vi "Teleop.vi"(10 "Match Info":T1={"Autonomous Elapsed Seconds"=0.0, "TeleOp Elapsed Seconds"=0.0, "Disabled Elapsed Seconds"=0.0, "Visited Autonomous"=FALSE, "Visited TeleOp"=FALSE, "Visited Disabled"=FALSE, "Autonomous Settings"={"Autonomous Style"=enum."Independent", "VI Refnum"=refnum}}, 11 "Call Context":T2) -> ()   [LabVIEW 2020]
doc: "This VI is called for each TeleOp packet received from the DS where the robot is not disabled. It is often used to read from the joysticks and update I/O or to update setpoints for timed control loops. It should complete and return within 20 milliseconds or it may miss DS packets."
uses:
  <vilib>/Rock Robotics/WPI/DriverStation/WPI_DriverStationDerivedRobotMode.ctl
  <vilib>/Rock Robotics/WPI/DriverStation/WPI_DriverStationMatch Info.ctl
  <vilib>/Rock Robotics/WPI/Joystick/XBox Axes Indexer.ctl
  <vilib>/Rock Robotics/WPI/ThirdParty/Phoenix-LabVIEW/Motor Controller/Controls/CTRE_Phoenix_MotorControl_ControlMode.ctl
  <vilib>/Rock Robotics/WPI/Utilities/WPI_GetSetVariantRefNum.vi
  <vilib>/Rock Robotics/Network Tables/NT Write Boolean Array.vi
  <vilib>/Rock Robotics/Network Tables/NT Write Numeric Array.vi
  <vilib>/Rock Robotics/Network Tables/NT Read Boolean.vi
  <vilib>/Rock Robotics/Network Tables/NT Read Number.vi
  <vilib>/Rock Robotics/WPI/ThirdParty/Phoenix-LabVIEW/Motor Controller/Get/CTRE_Phoenix_MotorController_GetSelectedSensorData.vi
panel:
  out "Voltage":dbl
  out "Sample Slider 0":dbl(slide) scale=0.0..5.0
  out "Sample Boolean 1":bool
  out "Sample Boolean 0":bool
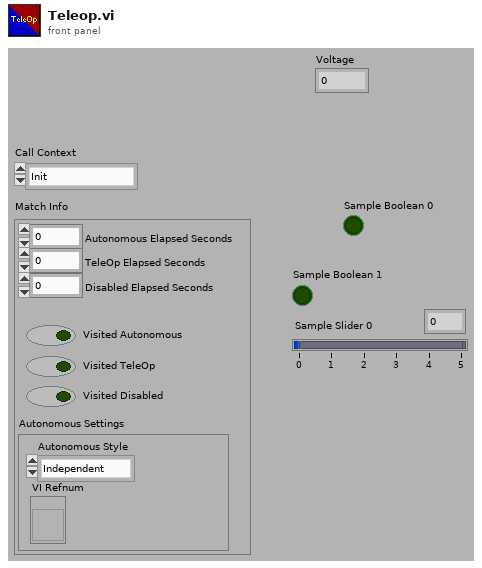
[diagram p1: front panel]
types:
  T1 = typedef "WPI_DriverStationMatch Info.ctl" = cluster{"Autonomous Elapsed Seconds":dbl, "TeleOp Elapsed Seconds":dbl, "Disabled Elapsed Seconds":dbl, "Visited Autonomous":bool, "Visited TeleOp":bool, "Visited Disabled":bool, "Autonomous Settings":cluster{"Autonomous Style":enum16{"Iterative", "Independent"}, "VI Refnum":refnum<vi>}}
  T2 = typedef "WPI_DriverStationDerivedRobotMode.ctl" = enum16{"Init", "Execute", "Stop"}
  T3 = typedef "CTRE_Phoenix_MotorControl_ControlMode.ctl" = u16
  T4 = typedef "XBox Axes Indexer.ctl" = enum16{"Left X", "Left Y", "Left Trigger", "Right Trigger", "Right X", "Right Y"}
  T5 = typedef "WPI_AnalogChannelDevRef.ctl" = cluster{"DevStatus":errorcluster, "Analog Channel":T6}
  T6 = typedef "FPGA_AIChannel.ctl" = enum8{"AI 0", "AI 1", "AI 2", "AI 3", "AI MXP 0", "AI MXP 1", "AI MXP 2", "AI MXP 3", "Invalid"}
  T7 = typedef "WPI_RobotDriveDevRef.ctl" = cluster{"DevStatus":errorcluster, "Motors[]":T8[], "Square Inputs":bool, "Max Output":dbl}
  T8 = typedef "WPI_MotorControlDeviceRef.ctl" = cluster{"DeviceStatus":errorcluster, "Type":T9, "PWM":cluster{"PWM Channel":T10, "DeadBand":T11}, "CAN":cluster{"Device Number":u8, "SetOutput VI Ref":variant, "GetOutput VI Ref":variant, "Enable VI Ref":variant, "Disable VI Ref":variant, "Data":variant}, "Invert":bool, "DIO PWM":cluster{"PWM \"Enable\" Channel":T10, "DIOChannel":T12, "PWM Rate":dbl}}
  T9 = typedef "WPI_MotorControlType.ctl" = enum16{"PWM", "CAN", "DIO PWM"}
  T10 = typedef "FPGA_DIOPWMChannel.ctl" = enum8{"PWM 0", "PWM 1", "PWM 2", "PWM 3", "PWM 4", "PWM 5", "PWM 6", "PWM 7", "PWM 8", "PWM 9", "PWM MXP 0", "PWM MXP 1", "PWM MXP 2", "PWM MXP 3", "PWM MXP 4", "PWM MXP 5", "PWM MXP 6", "PWM MXP 7", "PWM MXP 8", "PWM MXP 9", "Invalid"}
  T11 = typedef "WPI_PWMDeadband.ctl" = cluster{"Name":string, "maxPositivePwm":i32, "minPositivePwm":i32, "centerPwm":i32, "maxNegativePwm":i32, "minNegativePwm":i32, "angularRange":u16}
  T12 = typedef "FPGA_DIOChannel.ctl" = enum8{"DIO 0", "DIO 1", "DIO 2", "DIO 3", "DIO 4", "DIO 5", "DIO 6", "DIO 7", "DIO 8", "DIO 9", "DIO MXP 0", "DIO MXP 1", "DIO MXP 2", "DIO MXP 3", "DIO MXP 4", "DIO MXP 5", "DIO MXP 6", "DIO MXP 7", "DIO MXP 8", "DIO MXP 9", "DIO MXP 10", "DIO MXP 11", "DIO MXP 12", "DIO MXP 13", "DIO MXP 14", "DIO MXP 15", "SPI Port CS1", "SPI Port CS2", "SPI Port CS3", "SPI Port MISO", "SPI Port MOSI", "Invalid"}
  T13 = typedef "WPI_JoystickDevRef.ctl" = cluster{"Device":T14}
  T14 = typedef "WPI_JoystickDeviceEnum.ctl" = enum16{"USB 0", "USB 1", "USB 2", "USB 3", "USB 4", "USB 5"}
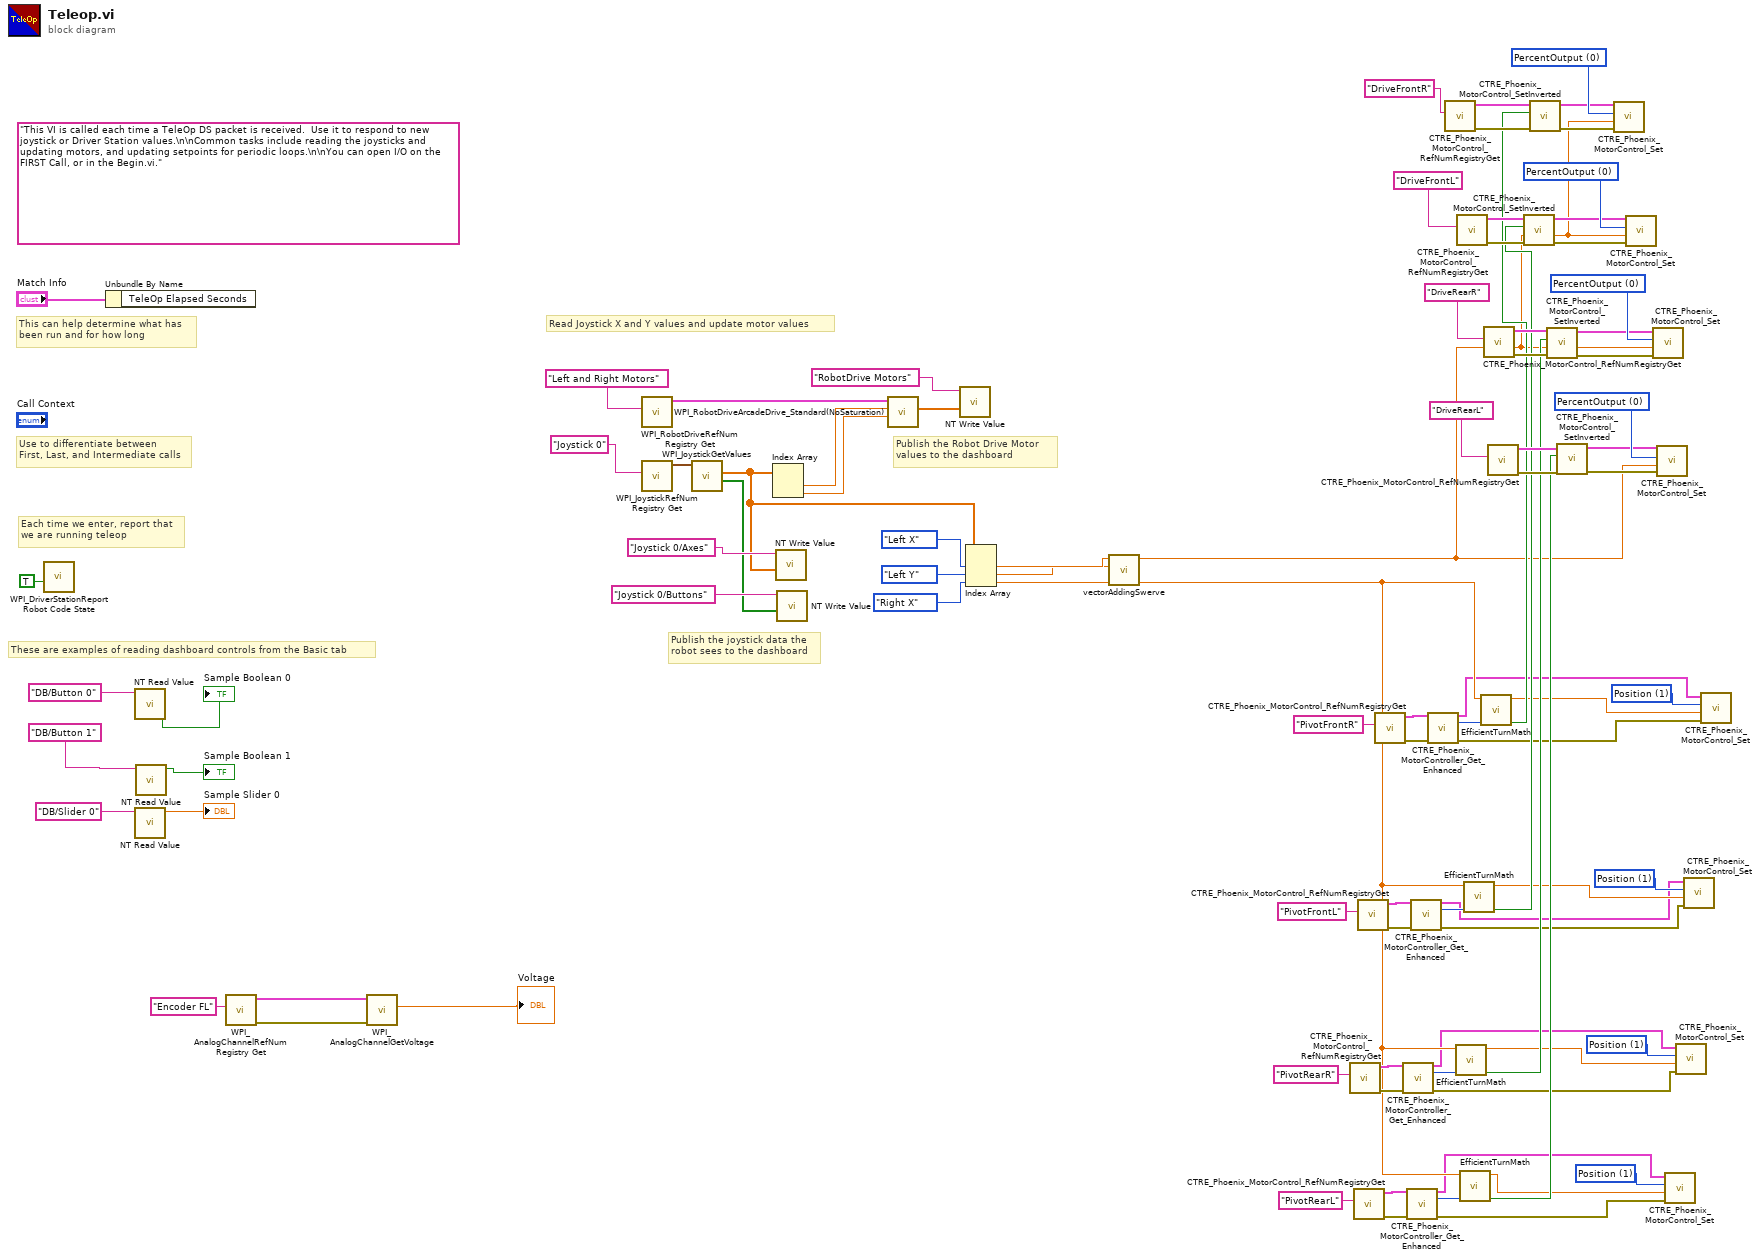
[diagram p0: block diagram]
diagram:
  w15 = T3 1 items=["PercentOutput"=0, "Position"=1, "Velocity"=2, "Current"=3, "Follower"=5, "MotionProfile"=6, "MotionMagic"=7, "MotionProfileArc"=10, "Disabled"=15] ("Control Mode")
  w16 = T3 1 items=["PercentOutput"=0, "Position"=1, "Velocity"=2, "Current"=3, "Follower"=5, "MotionProfile"=6, "MotionMagic"=7, "MotionProfileArc"=10, "Disabled"=15] ("Control Mode")
  w17 = T3 1 items=["PercentOutput"=0, "Position"=1, "Velocity"=2, "Current"=3, "Follower"=5, "MotionProfile"=6, "MotionMagic"=7, "MotionProfileArc"=10, "Disabled"=15] ("Control Mode")
  w19 = T3 1 items=["PercentOutput"=0, "Position"=1, "Velocity"=2, "Current"=3, "Follower"=5, "MotionProfile"=6, "MotionMagic"=7, "MotionProfileArc"=10, "Disabled"=15] ("Control Mode")
  w62 = T3 0 items=["PercentOutput"=0, "Position"=1, "Velocity"=2, "Current"=3, "Follower"=5, "MotionProfile"=6, "MotionMagic"=7, "MotionProfileArc"=10, "Disabled"=15] ("Control Mode")
  w63 = T3 0 items=["PercentOutput"=0, "Position"=1, "Velocity"=2, "Current"=3, "Follower"=5, "MotionProfile"=6, "MotionMagic"=7, "MotionProfileArc"=10, "Disabled"=15] ("Control Mode")
  w66 = T3 0 items=["PercentOutput"=0, "Position"=1, "Velocity"=2, "Current"=3, "Follower"=5, "MotionProfile"=6, "MotionMagic"=7, "MotionProfileArc"=10, "Disabled"=15] ("Control Mode")
  w67 = T3 0 items=["PercentOutput"=0, "Position"=1, "Velocity"=2, "Current"=3, "Follower"=5, "MotionProfile"=6, "MotionMagic"=7, "MotionProfileArc"=10, "Disabled"=15] ("Control Mode")
  (unwired) "This VI is called each time a TeleOp DS packet is received.  Use it to respond to new joystick or Driver Station values.\n\nCommon tasks include reading the joysticks and updating motors, and updating setpoints for periodic loops.\n\nYou can open I/O on the FIRST Call, or in the Begin.vi."
  # "These are examples of reading dashboard controls from the Basic tab"
  # "Publish the Robot Drive Motor\nvalues to the dashboard"
  # "Publish the joystick data the\nrobot sees to the dashboard"
  # "Each time we enter, report that\nwe are running teleop"
  # "Use to differentiate between\nFirst, Last, and Intermediate calls"
  # "This can help determine what has\nbeen run and for how long"
  # "Read Joystick X and Y values and update motor values"
  n1 = call <vilib>:"WPI_DriverStationReport Robot Code State.vi"("TeleOp"=TRUE ("Autonomous")) -> ()  [unwired: 10 in, 1 out]
  n2 = Unbundle By Name("Match Info") -> ()  [unwired: 1 out]
  n3 = call-poly <vilib>:"NT Read Value.vi"("Name"="DB/Button 0" ("refnum name")) -> ("Boolean"=→"Sample Boolean 0":bool)  [unwired: 9 in, 1 out]
  n4 = call-poly <vilib>:"NT Read Value.vi"("Name"="DB/Slider 0" ("refnum name")) -> ("Numeric"=→"Sample Slider 0":dbl)  [unwired: 9 in, 1 out]
  n5 = call-poly <vilib>:"NT Read Value.vi"("Name"="DB/Button 1" ("refnum name")) -> ("Boolean"=→"Sample Boolean 1":bool)  [unwired: 9 in, 1 out]
  n6 = call <vilib>:"WPI_AnalogChannelRefNum Registry Get.vi"("refnum name"="Encoder FL") -> ("error out"=w23:errorcluster, "AIDeviceRef"=w24:T5)  [unwired: 9 in]
  n7 = call <vilib>:"WPI_AnalogChannelGetVoltage.vi"("error in (no error)"=w23, "AIDeviceRef"=w24) -> ("Voltage"=→"Voltage":dbl)  [unwired: 7 in, 2 out]
  n8 = call <vilib>:"WPI_RobotDriveRefNum Registry Get.vi"("refnum name"="Left and Right Motors") -> ("RobotDriveDevRef"=w90:T7)  [unwired: 1 in, 9 out]
  n9 = call <vilib>:"WPI_JoystickRefNum Registry Get.vi"("refnum name"="Joystick 0") -> ("JoystickDevRef"=w87:T13)  [unwired: 1 in, 9 out]
  n10 = call <vilib>:"WPI_JoystickGetValues.vi"("JoystickDevRef"=w87) -> ("Buttons"=w82:bool[], "Axes"=w73:dbl[])  [unwired: 6 in, 3 out]
  n11 = Index Array(array=w73) -> (element #1=w89:dbl, element #2=w85:dbl)  [unwired: 2 in]
  n12 = call-poly <vilib>:"NT Write Value.vi"("Numeric Array"=w73, "Name"="Joystick 0/Axes") -> ()  [unwired: 9 in, 1 out]
  n13 = call-poly <vilib>:"NT Write Value.vi"("Boolean Array"=w82, "Name"="Joystick 0/Buttons") -> ()  [unwired: 9 in, 1 out]
  n14 = call <vilib>:"WPI_RobotDriveArcadeDrive_Standard(NoSaturation).vi"("Y axis value"=w85, "X axis value"=w89, "RobotDriveDevRef"=w90) -> ("Motor Values"=w75:dbl[])  [unwired: 1 in, 7 out]
  n15 = call-poly <vilib>:"NT Write Value.vi"("Numeric Array"=w75, "Name"="RobotDrive Motors") -> ()  [unwired: 9 in, 1 out]
  n16 = Index Array(array=w73, index #1=XBox_Axes_Indexer."Left X" ("XBox Axes"), index #2=XBox_Axes_Indexer."Left Y" ("XBox Axes"), index #3=XBox_Axes_Indexer."Right X" ("XBox Axes")) -> (element #1=w3:dbl, element #2=w1:dbl, element #3=w2:dbl)
  n17 = call "vectorAddingSwerve.vi"("RightX"=w2, "LeftY"=w1, "LeftX"=w3) -> ("Magnitude"=w20:dbl, "Speed"=w21:dbl)  [unwired: 7 in]
  n18 = call <vilib>:"CTRE_Phoenix_MotorControl_RefNumRegistryGet.vi"("refnum name"="PivotRearR") -> ("error out"=w37:errorcluster, "PhoenixMotorControlDevRef"=w36:T8)  [unwired: 9 in]
  n19 = call <vilib>:"CTRE_Phoenix_MotorControl_RefNumRegistryGet.vi"("refnum name"="PivotRearL") -> ("error out"=w40:errorcluster, "PhoenixMotorControlDevRef"=w41:T8)  [unwired: 9 in]
  n20 = call <vilib>:"CTRE_Phoenix_MotorControl_RefNumRegistryGet.vi"("refnum name"="PivotFrontL") -> ("error out"=w43:errorcluster, "PhoenixMotorControlDevRef"=w44:T8)  [unwired: 9 in]
  n21 = call <vilib>:"CTRE_Phoenix_MotorControl_RefNumRegistryGet.vi"("refnum name"="PivotFrontR") -> ("error out"=w34:errorcluster, "PhoenixMotorControlDevRef"=w33:T8)  [unwired: 9 in]
  n22 = call-poly <vilib>:"CTRE_Phoenix_MotorController_Get_Enhanced.vi"("PhoenixMotorControlDevRef"=w36, "error in"=w37) -> ("PhoenixMotorControlDevRef"=w9:T8, "Position (Raw Sensor Units)"=w38:i32, "error out"=w7:errorcluster)  [unwired: 10 in, 1 out]
  n23 = call-poly <vilib>:"CTRE_Phoenix_MotorController_Get_Enhanced.vi"("PhoenixMotorControlDevRef"=w41, "error in"=w40) -> ("PhoenixMotorControlDevRef"=w8:T8, "Position (Raw Sensor Units)"=w39:i32, "error out"=w4:errorcluster)  [unwired: 10 in, 1 out]
  n24 = call-poly <vilib>:"CTRE_Phoenix_MotorController_Get_Enhanced.vi"("PhoenixMotorControlDevRef"=w44, "error in"=w43) -> ("PhoenixMotorControlDevRef"=w10:T8, "Position (Raw Sensor Units)"=w42:i32, "error out"=w6:errorcluster)  [unwired: 10 in, 1 out]
  n25 = call-poly <vilib>:"CTRE_Phoenix_MotorController_Get_Enhanced.vi"("PhoenixMotorControlDevRef"=w33, "error in"=w34) -> ("PhoenixMotorControlDevRef"=w11:T8, "Position (Raw Sensor Units)"=w35:i32, "error out"=w5:errorcluster)  [unwired: 10 in, 1 out]
  n26 = call <vilib>:"CTRE_Phoenix_MotorControl_RefNumRegistryGet.vi"("refnum name"="DriveFrontR") -> ("error out"=w46:errorcluster, "PhoenixMotorControlDevRef"=w48:T8)  [unwired: 9 in]
  n27 = call "EfficientTurnMath.vi"("current"=w38, "target"=w20) -> ("Invert"=w26:bool, "AngleToTurn"=w12:dbl)  [unwired: 8 in]
  n28 = call <vilib>:"CTRE_Phoenix_MotorControl_RefNumRegistryGet.vi"("refnum name"="DriveFrontL") -> ("error out"=w50:errorcluster, "PhoenixMotorControlDevRef"=w52:T8)  [unwired: 9 in]
  n29 = call "EfficientTurnMath.vi"("current"=w39, "target"=w20) -> ("Invert"=w27:bool, "AngleToTurn"=w18:dbl)  [unwired: 8 in]
  n30 = call "EfficientTurnMath.vi"("current"=w42, "target"=w20) -> ("Invert"=w28:bool, "AngleToTurn"=w13:dbl)  [unwired: 8 in]
  n31 = call "EfficientTurnMath.vi"("current"=w35, "target"=w20) -> ("Invert"=w25:bool, "AngleToTurn"=w14:dbl)  [unwired: 8 in]
  n32 = call <vilib>:"CTRE_Phoenix_MotorControl_RefNumRegistryGet.vi"("refnum name"="DriveRearR") -> ("error out"=w54:errorcluster, "PhoenixMotorControlDevRef"=w56:T8)  [unwired: 9 in]
  n33 = call <vilib>:"CTRE_Phoenix_MotorControl_RefNumRegistryGet.vi"("refnum name"="DriveRearL") -> ("error out"=w59:errorcluster, "PhoenixMotorControlDevRef"=w60:T8)  [unwired: 9 in]
  n34 = call <vilib>:"CTRE_Phoenix_MotorControl_SetInverted.vi"("error in (no error)"=w50, "Invert?"=w28, "PhoenixMotorControlDevRef"=w52) -> ("error out"=w49:errorcluster, "PhoenixMotorControlDevRef"=w51:T8)  [unwired: 7 in]
  n35 = call <vilib>:"CTRE_Phoenix_MotorControl_SetInverted.vi"("error in (no error)"=w46, "Invert?"=w25, "PhoenixMotorControlDevRef"=w48) -> ("error out"=w45:errorcluster, "PhoenixMotorControlDevRef"=w47:T8)  [unwired: 7 in]
  n36 = call <vilib>:"CTRE_Phoenix_MotorControl_SetInverted.vi"("error in (no error)"=w54, "Invert?"=w26, "PhoenixMotorControlDevRef"=w56) -> ("error out"=w53:errorcluster, "PhoenixMotorControlDevRef"=w55:T8)  [unwired: 7 in]
  n37 = call <vilib>:"CTRE_Phoenix_MotorControl_SetInverted.vi"("error in (no error)"=w59, "Invert?"=w27, "PhoenixMotorControlDevRef"=w60) -> ("error out"=w57:errorcluster, "PhoenixMotorControlDevRef"=w58:T8)  [unwired: 7 in]
  n38 = call <vilib>:"CTRE_Phoenix_MotorControl_Set.vi"("error in (no error)"=w45, "Output"=w21, "Control Mode"=w62, "PhoenixMotorControlDevRef"=w47) -> ()  [unwired: 6 in, 2 out]
  n39 = call <vilib>:"CTRE_Phoenix_MotorControl_Set.vi"("error in (no error)"=w49, "Output"=w21, "Control Mode"=w63, "PhoenixMotorControlDevRef"=w51) -> ()  [unwired: 6 in, 2 out]
  n40 = call <vilib>:"CTRE_Phoenix_MotorControl_Set.vi"("error in (no error)"=w53, "Output"=w21, "Control Mode"=w66, "PhoenixMotorControlDevRef"=w55) -> ()  [unwired: 6 in, 2 out]
  n41 = call <vilib>:"CTRE_Phoenix_MotorControl_Set.vi"("error in (no error)"=w57, "Output"=w21, "Control Mode"=w67, "PhoenixMotorControlDevRef"=w58) -> ()  [unwired: 6 in, 2 out]
  n42 = call <vilib>:"CTRE_Phoenix_MotorControl_Set.vi"("error in (no error)"=w4, "Output"=w18, "Control Mode"=w19, "PhoenixMotorControlDevRef"=w8) -> ()  [unwired: 6 in, 2 out]
  n43 = call <vilib>:"CTRE_Phoenix_MotorControl_Set.vi"("error in (no error)"=w7, "Output"=w12, "Control Mode"=w17, "PhoenixMotorControlDevRef"=w9) -> ()  [unwired: 6 in, 2 out]
  n44 = call <vilib>:"CTRE_Phoenix_MotorControl_Set.vi"("error in (no error)"=w6, "Output"=w13, "Control Mode"=w16, "PhoenixMotorControlDevRef"=w10) -> ()  [unwired: 6 in, 2 out]
  n45 = call <vilib>:"CTRE_Phoenix_MotorControl_Set.vi"("error in (no error)"=w5, "Output"=w14, "Control Mode"=w15, "PhoenixMotorControlDevRef"=w11) -> ()  [unwired: 6 in, 2 out]
